vi "In progress 1.vi"   [LabVIEW 2013]
types:
  T1 = typedef "WPI_EncoderDevRef.ctl" = cluster{"DevStatus":errorcluster, "EncoderIndex":T2, "CounterIndex":T3, "DistancePerCount":dbl, "Decoding Type":T4}
  T2 = typedef "FPGA_EncoderIdx.ctl" = enum8{"Enc 0", "Enc 1", "Enc 2", "Enc 3", "Invalid"}
  T3 = typedef "FPGA_CounterCtrSystemIndex.ctl" = enum8{"Ctr 0", "Ctr 1", "Ctr 2", "Ctr 3", "Ctr 4", "Ctr 5", "Ctr 6", "Ctr 7", "Invalid"}
  T4 = typedef "WPI_EncoderType.ctl" = enum16{"1x", "2x", "4x"}
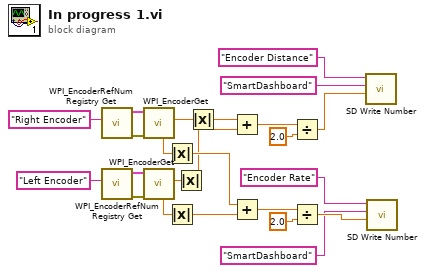
[diagram p0: block diagram]
diagram:
  n1 = call <vilib>:"WPI_EncoderRefNum Registry Get.vi"("refnum name"="Right Encoder") -> ("error out"=w16:errorcluster, "EncoderDevRef"=w17:T1)  [unwired: 9 in]
  n2 = call <vilib>:"WPI_EncoderRefNum Registry Get.vi"("refnum name"="Left Encoder") -> ("error out"=w19:errorcluster, "EncoderDevRef"=w18:T1)  [unwired: 9 in]
  n3 = call <vilib>:"WPI_EncoderGet.vi"("error in (no error)"=w16, "EncoderDevRef"=w17) -> ("Distance"=w7:dbl, "Rate"=w23:dbl)  [unwired: 4 in, 4 out]
  n4 = call <vilib>:"WPI_EncoderGet.vi"("error in (no error)"=w19, "EncoderDevRef"=w18) -> ("Distance"=w6:dbl, "Rate"=w24:dbl)  [unwired: 4 in, 4 out]
  n5 = Absolute Value(x=w23) -> (abs(x)=w4:dbl)
  n6 = Absolute Value(x=w24) -> (abs(x)=w3:dbl)
  n7 = Absolute Value(x=w6) -> (abs(x)=w2:dbl)
  n8 = Absolute Value(x=w7) -> (abs(x)=w1:dbl)
  n9 = Add(x=w1, y=w2) -> (x+y=w9:dbl)
  n10 = Add(x=w4, y=w3) -> (x+y=w21:dbl)
  n11 = Divide(x=w9, y=2.0) -> (x/y=w5:dbl)
  n12 = Divide(x=w21, y=2.0) -> (x/y=w14:dbl)
  n13 = call <vilib>:"SD Write Number.vi"("Numeric"=w5, "Table Prefix"="SmartDashboard", "Name"="Encoder Distance") -> ()  [unwired: 7 in, 2 out]
  n14 = call <vilib>:"SD Write Number.vi"("Numeric"=w14, "Table Prefix"="SmartDashboard", "Name"="Encoder Rate") -> ()  [unwired: 7 in, 2 out]
